vi "Error Test Number Of Bits.vi"(8 "error in":errorcluster, 10 "number of bits":i32) -> (0 "error out":errorcluster)   [LabVIEW 2020, in "Ballard ARINC 429 Import.lvlib"]
uses:
  Ballard ARINC 429 Import.lvlib
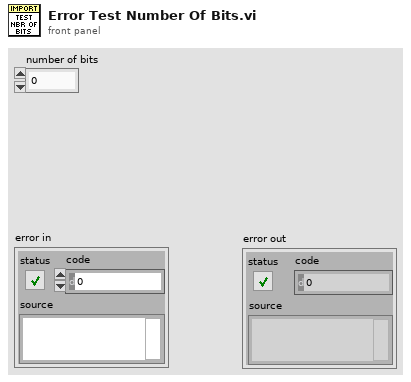
[diagram p1: front panel]
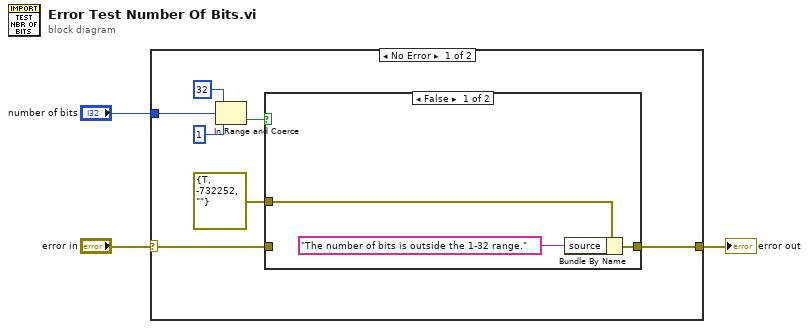
[diagram p0: block diagram]
diagram:
  n1 = case shown="No Error" "error in" {
    selector: "error in" -> [w9 w15]
    tunnel: [w8 w15] -> w2
    tunnel: "number of bits" -> [w10 _]
    frame No Error {
      n2 = In Range and Coerce(upper limit=32 ("lower limit"), x=w10, lower limit=1) -> (In Range?=w4:bool)  [unwired: 1 out]
      n3 = case shown="False" w4 {
        tunnel: w9 -> [_ w14]
        tunnel: [w12 w14] -> w8
        tunnel: errorcluster {"status"=TRUE, "code"=-732252, "source"=""} ("error constant") -> [w13 _]
        frame False {
          n4 = Bundle By Name(cluster=w13, "source"="The number of bits is outside the 1-32 range.") -> (w12:errorcluster)
        }
        frame True {
        }
      }
    }
    frame Error {
    }
  }
  "error out" <- w2
